vi "f_corr(SubVI).vi"(9 "m":dbl, 10 "Gaussian noise pattern 2":dbl[](array[numeric]), 11 "Gaussian noise pattern":dbl[](array[numeric])) -> (3 "f_corr":dbl)   [LabVIEW 2025]
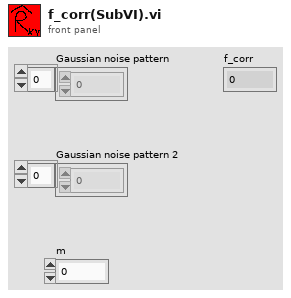
[diagram p1: front panel]
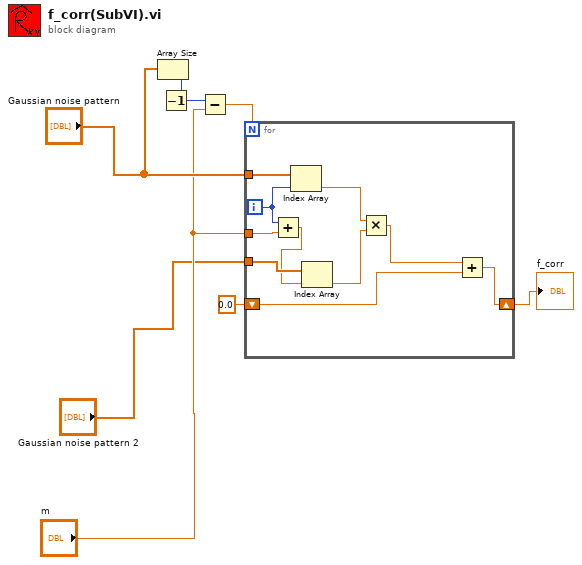
[diagram p0: block diagram]
diagram:
  n1 = Array Size(array="Gaussian noise pattern") -> (size(s)=w7:i32)
  n2 = Decrement(x=w7) -> (x-1=w2:i32)
  n3 = Subtract(x=w2, y="m") -> (x-y=w1:dbl)
  n4 = for {
    N: w1 -> [_]
    tunnel: "Gaussian noise pattern" -> [w18]
    tunnel: "Gaussian noise pattern 2" -> [w17]
    tunnel: "m" -> [w15]
    shift-right: [w11] -> w6
    shift-left: 0.0 -> [w9]
    i -> [w14]
    n5 = Add(x=w14, y=w15) -> (x+y=w13:dbl)
    n6 = Index Array(array=w18, index=w14) -> (element=w16:dbl)
    n7 = Index Array(array=w17, index=w13) -> (element=w12:dbl)
    n8 = Multiply(x=w16, y=w12) -> (x*y=w10:dbl)
    n9 = Add(x=w10, y=w9) -> (x+y=w11:dbl)
  }
  "f_corr" <- w6
